vi "_Obsolete_PathPlanner_Path_JoinPaths.vi"(11 "in Trajectories":T1[](array[typedef]) {"States"."TargetHolonomicRotation"."SIN" format="%13.4f"; "States"."TargetHolonomicRotation"."COS" format="%13.4f"; "States"."TargetHolonomicRotation"."VALUE" format="%13.4f"; "States"."Heading"."SIN" format="%13.4f"; "States"."Heading"."COS" format="%13.4f"; "States"."Heading"."VALUE" format="%13.4f"; "States"."PositionMeters"."Y" format="%14.3f"; "States"."PositionMeters"."X" format="%14.3f"}) -> (3 "out PathPlannerTrajectory":T1 {"States"."TargetHolonomicRotation"."SIN" format="%13.4f"; "States"."TargetHolonomicRotation"."COS" format="%13.4f"; "States"."TargetHolonomicRotation"."VALUE" format="%13.4f"; "States"."Heading"."SIN" format="%13.4f"; "States"."Heading"."COS" format="%13.4f"; "States"."Heading"."VALUE" format="%13.4f"; "States"."PositionMeters"."Y" format="%14.3f"; "States"."PositionMeters"."X" format="%14.3f"})   [LabVIEW 2019, in "PathPlanner24.lvlib"]
uses:
  PathPlanner24.lvlib
  TypeDef/PathPlannerTrajectory.ctl
  TypeDef/PathPlannerTrajectoryState.ctl
  <vilib>/Rock Robotics/WPI/ThirdParty/JAS_Junk/TrajLib/TypeDef/TRANSLATION2D.ctl
  <vilib>/Rock Robotics/WPI/ThirdParty/JAS_Junk/TrajLib/TypeDef/ROTATION2D.ctl
  TypeDef/PathPlannerPathConstraints.ctl
  <vilib>/Rock Robotics/WPI/ThirdParty/JAS_Junk/TrajLib/Trajectory_Library.lvlib
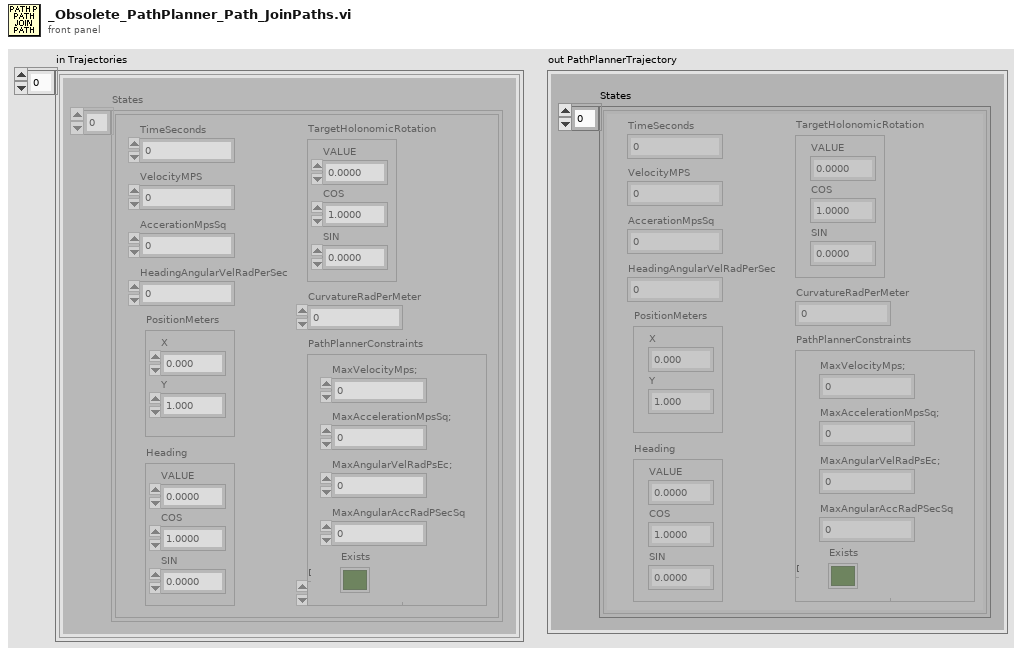
[diagram p1: front panel]
types:
  T1 = typedef "PathPlanner24.lvlib/PathPlannerTrajectory.ctl" = cluster{"States":T2[]}
  T2 = typedef "PathPlanner24.lvlib/PathPlannerTrajectoryState.ctl" = cluster{"TimeSeconds":dbl, "VelocityMPS":dbl, "AccerationMpsSq":dbl, "HeadingAngularVelRadPerSec":dbl, "PositionMeters":T3, "Heading":T4, "TargetHolonomicRotation":T4, "CurvatureRadPerMeter":dbl, "DeltaPos":dbl, "PathPlannerConstraints":T5}
  T3 = typedef "Trajectory_Library.lvlib/TRANSLATION2D.ctl" = cluster{"X":dbl, "Y":dbl}
  T4 = typedef "Trajectory_Library.lvlib/ROTATION2D.ctl" = cluster{"VALUE":dbl, "COS":dbl, "SIN":dbl}
  T5 = typedef "PathPlanner24.lvlib/PathPlannerPathConstraints.ctl" = cluster{"MaxVelocityMps;":dbl, "MaxAccelerationMpsSq;":dbl, "MaxAngularVelRadPsEc;":dbl, "MaxAngularAccRadPSecSq":dbl, "Exists":bool}
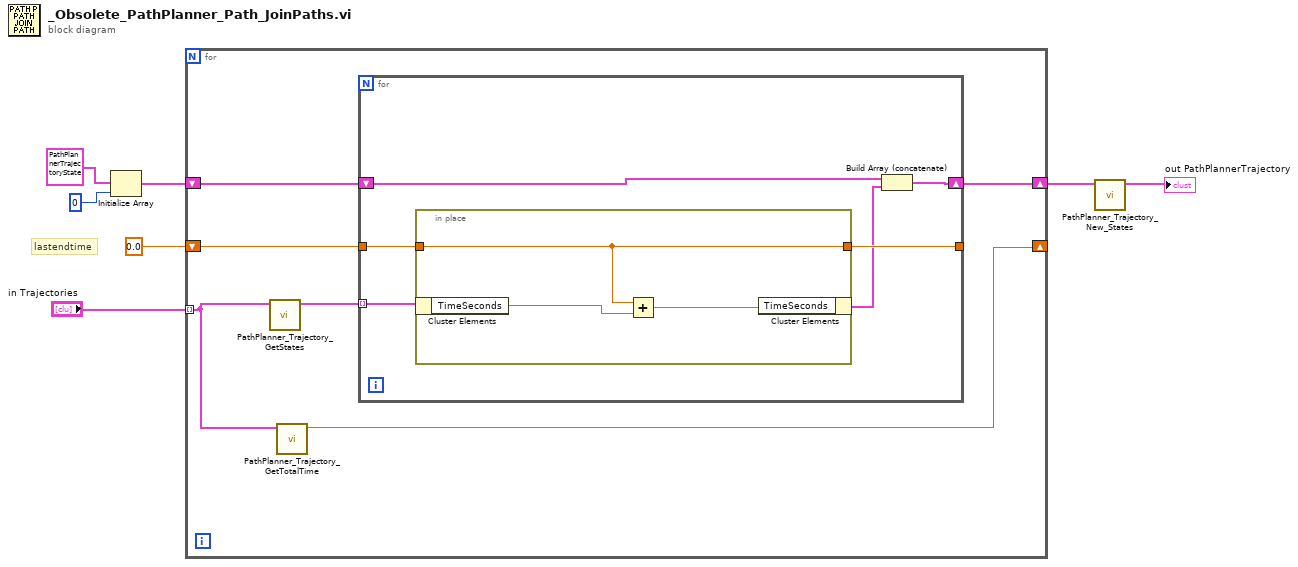
[diagram p0: block diagram]
diagram:
  # "lastendtime"
  n1 = Initialize Array(T2 {"TimeSeconds"=0.0, "VelocityMPS"=0.0, "AccerationMpsSq"=0.0, "HeadingAngularVelRadPerSec"=0.0, "PositionMeters"={"X"=0.0, "Y"=1.0}, "Heading"={"VALUE"=0.0, "COS"=1.0, "SIN"=0.0}, "TargetHolonomicRotation"={"VALUE"=0.0, "COS"=1.0, "SIN"=0.0}, "CurvatureRadPerMeter"=0.0, "DeltaPos"=0.0, "PathPlannerConstraints"={"MaxVelocityMps;"=0.0, "MaxAccelerationMpsSq;"=0.0, "MaxAngularVelRadPsEc;"=0.0, "MaxAngularAccRadPSecSq"=0.0, "Exists"=FALSE}} ("PathPlannerState"), 0 ("dimension size")) -> (w5:T2[])
  n2 = for {
    shift-right: [w11] -> w2
    shift-left: w5 -> [w12]
    shift-right: [w10] -> _
    shift-left: 0.0 -> [w13]
    tunnel: "in Trajectories" -> [w9] mode=indexing
    n3 = call "PathPlanner_Trajectory_GetStates.vi"("PathPlannerTrajectory"=w9) -> ("PathPlannerStates"=w8:T2[])  [unwired: 10 in]
    n4 = call "PathPlanner_Trajectory_GetTotalTime.vi"("PathPlannerTrajectory"=w9) -> ("TotalTimeSeconds"=w10:dbl)  [unwired: 10 in]
    n5 = for {
      tunnel: w8 -> [w19] mode=indexing
      tunnel: w13 -> [w18]
      tunnel: [w17] -> _
      shift-right: [w14] -> w11
      shift-left: w12 -> [w15]
      n6 = in-place {
        in-place-border: w18 -> [w20]
        in-place-border: [w20] -> w17
        n7 = in-place-cluster #1(w19) -> ("TimeSeconds"=w21:dbl)
        n8 = Add(x=w20, y=w21) -> (x+y=w22:dbl)
        n9 = in-place-cluster #1("TimeSeconds"=w22) -> (w16:T2)
      }
      n10 = Build Array (concatenate)(w15, w16) -> (w14:T2[])
    }
  }
  n11 = call "PathPlanner_Trajectory_New_States.vi"("PathPlannerStates"=w2) -> ("PathPlannerTrajectory"=→"out PathPlannerTrajectory":T1)  [unwired: 10 in]
